vi "DAQ Mean Data UI.vi"() -> ()   [LabVIEW 2016]
uses:
  <vilib>/Utility/miscctls.llb/LVRowAndColumnTypeDef.ctl
  X-DAQ Viewer/Controls/ConfigFGVCtrl.ctl
  Ctrls/GlobeVaribles.vi
  Architecture/Queue Management/ARC_Queue Valid.vi
panel:
  out "Table":string[][](table)
  in  "Caller":string
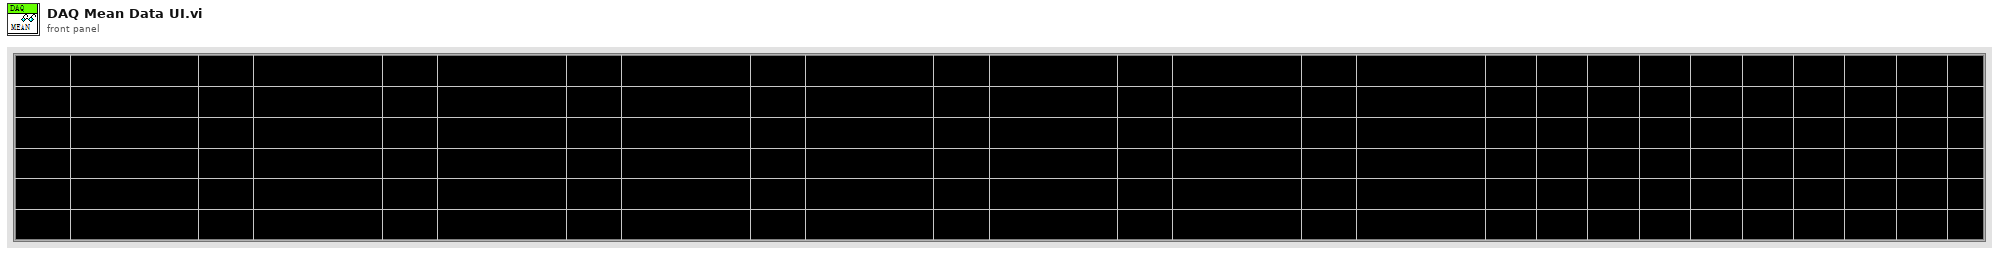
[diagram p1: front panel]
types:
  T1 = typedef "LVRowAndColumnTypeDef.ctl" = cluster{"Row":i32, "Column":i32}
  T2 = typedef "ConfigFGVCtrl.ctl" = enum16{"Initialize", "Get Value", "Set Value", "Search Info"}
  T3 = typedef "HardWare _ Channel Info.ctl" = cluster{"PhyCHtags[]":string[], "VCHTags":string[], "AllNames":string[], "AllAlias":string[], "AllUnits":string[], "AllName(Unit)":string[], "AllAlarmMax":dbl[], "AllAlarmMin":dbl[], "VCHFormula[]":string[], "VCHAlias[]":string[]}
  T4 = typedef "Continuous Operations.ctl" = enum16{"Writting", "Pause", "Stop"}
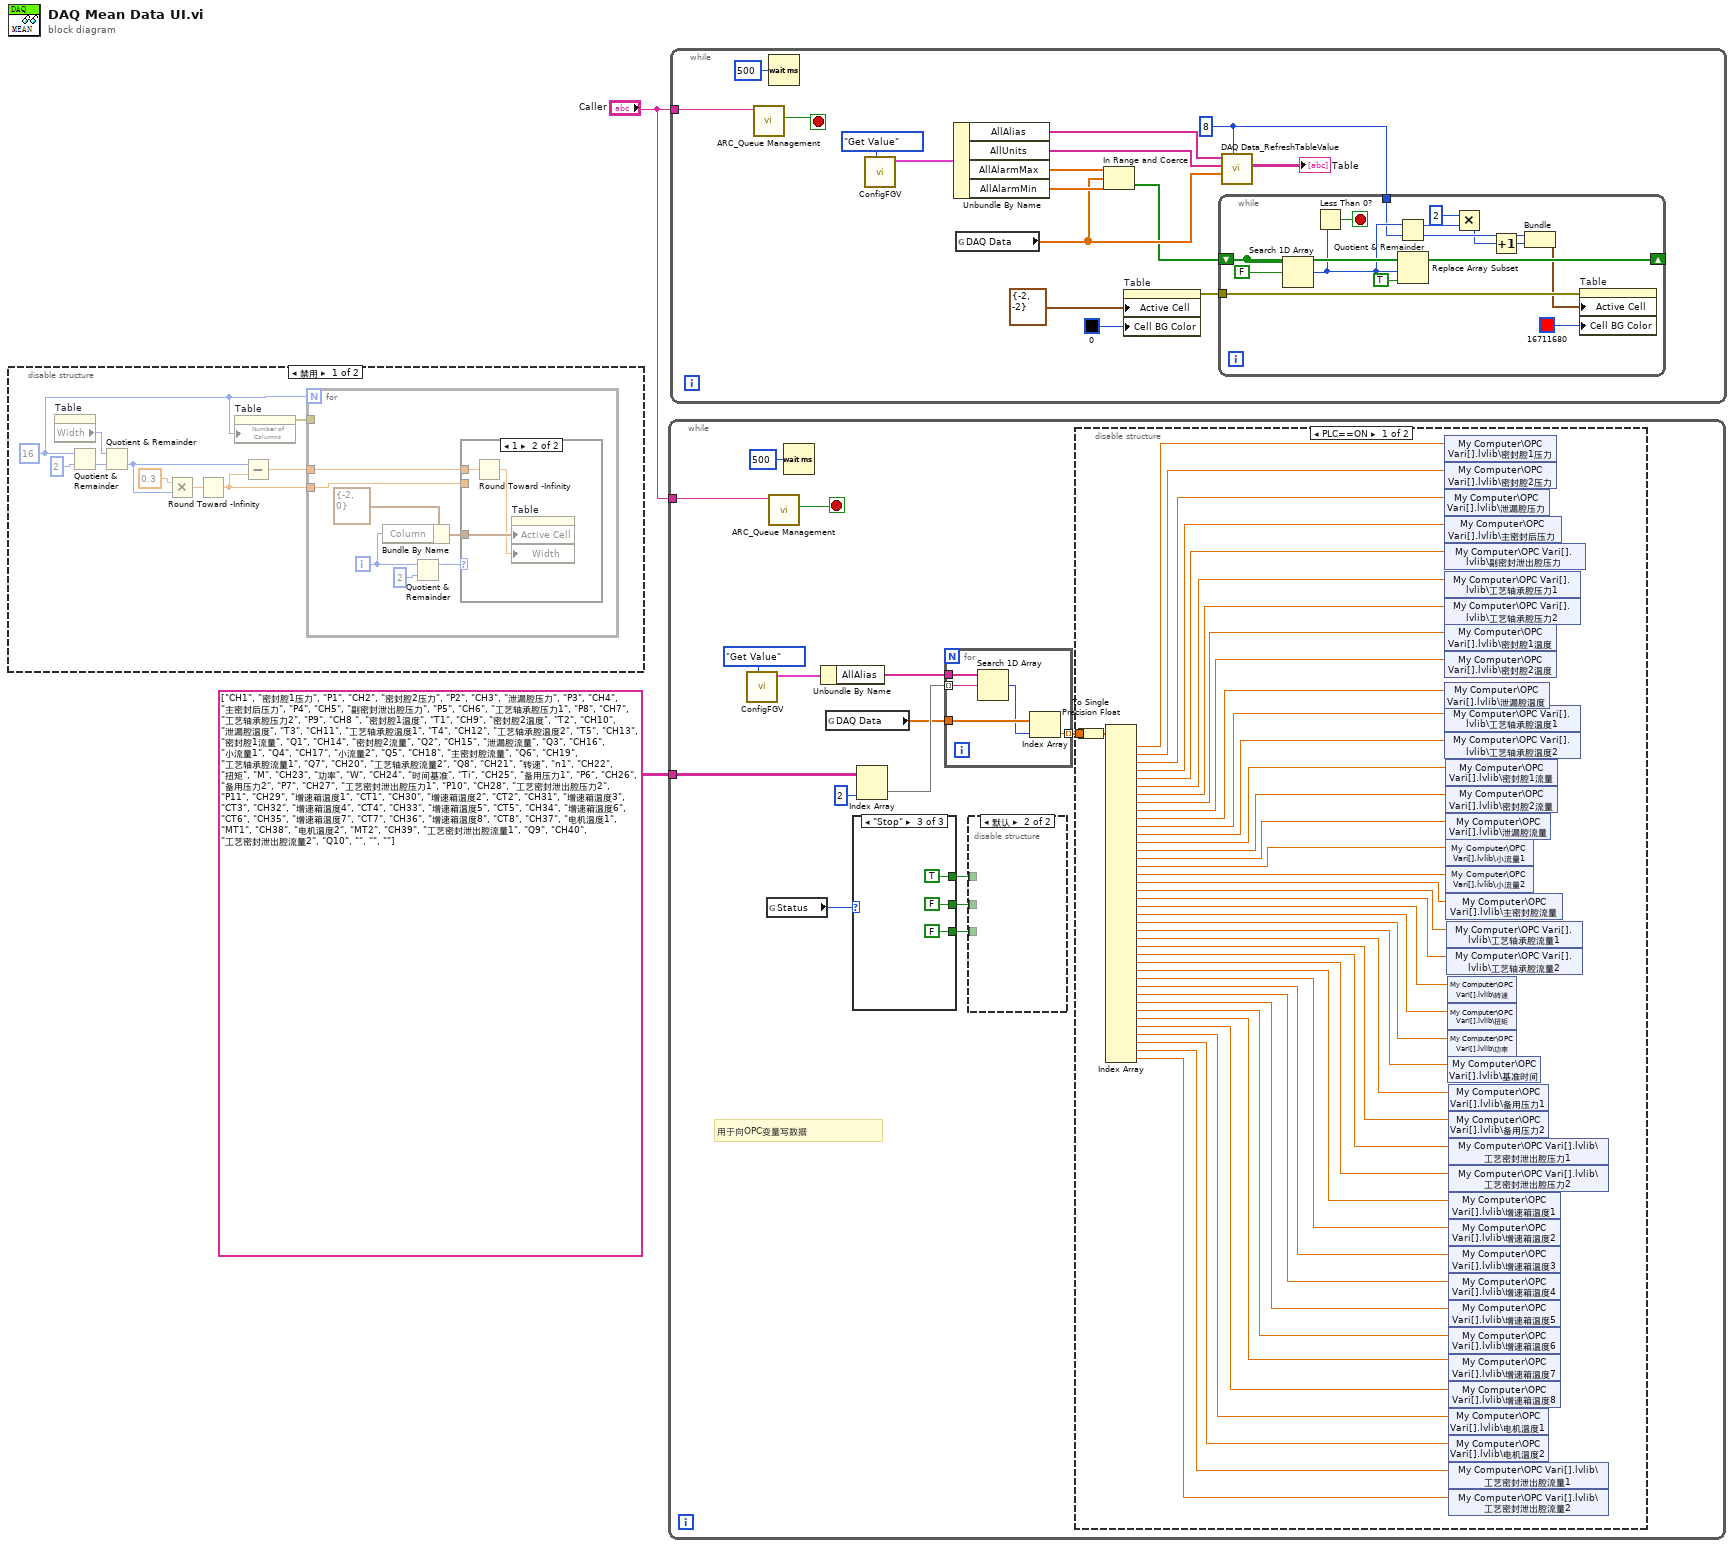
[diagram p0: block diagram]
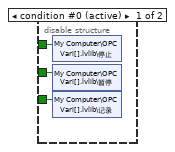
[diagram p2: hidden frame]
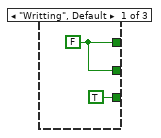
[diagram p4: hidden frame]
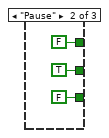
[diagram p5: hidden frame]
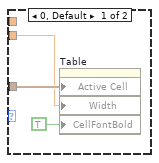
[diagram p6: hidden frame]
diagram:
  n1 = disable-structure shown="禁用" {
    frame Disabled {
      w4 = 16
      n2 = property on="Table" class="Tbl (strict)"() -> ("Width"=w9:u32)  [unwired: 2 in, 2 out]
      n3 = Quotient & Remainder(x=w4, y=2) -> (floor(x/y)=w11:i32)  [unwired: 1 out]
      n4 = Quotient & Remainder(x=w9, y=w11) -> (floor(x/y)=w6:u32)  [unwired: 1 out]
      n5 = Multiply(x=0.3, y=w6) -> (x*y=w8:dbl)
      n6 = Round Toward -Infinity(1:w8) -> (0:w5:dbl)
      n7 = property on="Table" class="Tbl (strict)"("Number of Columns"=w4) -> (error out=w3:errorcluster)  [unwired: 2 in, 1 out]
      n8 = Subtract(x=w6, y=w5) -> (x-y=w7:dbl)
      n9 = for {
        N: w4 -> [_]
        tunnel: w5 -> [w14]
        tunnel: w7 -> [w13]
        tunnel: w3 -> [_]
        i -> [w17]
        n10 = Bundle By Name(cluster=T1 {"Row"=-2, "Column"=0} ("活动单元格:活动单元格"), "Column"=w17) -> (w18:T1)
        n11 = Quotient & Remainder(x=w17, y=2) -> (x-y*floor(x/y)=w15:i32)  [unwired: 1 out]
        n12 = case shown="1" w15 {
          tunnel: w18 -> [w22 w25]
          tunnel: w14 -> [w20 _]
          tunnel: w13 -> [_ w24]
          frame 0, Default {
            n13 = property on="Table" class="Tbl (strict)"("Active Cell"=w22, "Width"=w20, "CellFontBold"=TRUE ("活动单元格:单元格字体:粗体")) -> ()  [unwired: 2 in, 2 out]
          }
          frame 1 {
            n14 = Round Toward -Infinity(1:w24) -> (0:w23:dbl)
            n15 = property on="Table" class="Tbl (strict)"("Active Cell"=w25, "Width"=w23) -> ()  [unwired: 2 in, 2 out]
          }
        }
      }
    }
    frame Enabled {
    }
  }
  n16 = while {
    tunnel: "Caller" -> [w39]
    tunnel: string[][] [["CH1", "密封腔1压力", "P1"], ["CH2", "密封腔2压力", "P2"], ["CH3", "泄漏腔压力", "P3"], ["CH4", "主密封后压力", "P4"], ["CH5", "副密封泄出腔压力", "P5"], ["CH6", "工艺轴承腔压力1", "P8"], ["CH7", "工艺轴承腔压力2", "P9"], ["CH8 ", "密封腔1温度", "T1"], ["CH9", "密封腔2温度", "T2"], ["CH10", "泄漏腔温度", "T3"], ["CH11", "工艺轴承腔温度1", "T4"], ["CH12", "工艺轴承腔温度2", "T5"], ["CH13", "密封腔1流量", "Q1"], ["CH14", "密封腔2流量", "Q2"], ["CH15", "泄漏腔流量", "Q3"], ["CH16", "小流量1", "Q4"], ["CH17", "小流量2", "Q5"], ["CH18", "主密封腔流量", "Q6"], ["CH19", "工艺轴承腔流量1", "Q7"], ["CH20", "工艺轴承腔流量2", "Q8"], ["CH21", "转速", "n1"], ["CH22", "扭矩", "M"], ["CH23", "功率", "W"], ["CH24", "时间基准", "Ti"], ["CH25", "备用压力1", "P6"], ["CH26", "备用压力2", "P7"], ["CH27", "工艺密封泄出腔压力1", "P10"], ["CH28", "工艺密封泄出腔压力2", "P11"], ["CH29", "增速箱温度1", "CT1"], ["CH30", "增速箱温度2", "CT2"], ["CH31", "增速箱温度3", "CT3"], ["CH32", "增速箱温度4", "CT4"], ["CH33", "增速箱温度5", "CT5"], ["CH34", "增速箱温度6", "CT6"], ["CH35", "增速箱温度7", "CT7"], ["CH36", "增速箱温度8", "CT8"], ["CH37", "电机温度1", "MT1"], ["CH38", "电机温度2", "MT2"], ["CH39", "工艺密封泄出腔流量1", "Q9"], ["CH40", "工艺密封泄出腔流量2", "Q10"], ["", "", ""]] ("数组") -> [w35]
    stop <- w38 stop-if-true
    # "用于向OPC变量写数据"
    n17 = call "ConfigFGV.vi"("Command"=ConfigFGVCtrl."Get Value") -> ("CHInfoOut"=w37:T3)  [unwired: 6 in, 4 out]
    n18 = global read "GlobeVaribles.vi" "Status"() -> (w29:T4)
    n19 = call-poly "ARC_Queue Management.vi"("Queue Name(unamed)"=w39) -> ("Not Exist?"=w38:bool)  [unwired: 8 in, 2 out]
    n20 = Wait (ms)(milliseconds to wait=u32 500 ("等待时间（毫秒）")) -> ()  [unwired: 1 out]
    n21 = Unbundle By Name(w37) -> ("AllAlias"=w33:string[])
    n22 = global read "GlobeVaribles.vi" "DAQ Data"() -> (w31:dbl[])
    n23 = case shown="\"Stop\"" w29 {
      tunnel: [w87 FALSE TRUE] -> w28
      tunnel: [w87 TRUE FALSE] -> w27
      tunnel: [TRUE FALSE FALSE] -> w26
      frame "Writting", Default {
        w87 = FALSE
      }
      frame "Pause" {
      }
      frame "Stop" {
      }
    }
    n24 = Index Array(array=w35, index (col)=2 ("禁用的索引 (列)")) -> (element=w32:string[])  [unwired: 1 in]
    n25 = for {
      tunnel: w33 -> [w98]
      tunnel: w32 -> [w97] mode=indexing
      tunnel: w31 -> [w96]
      tunnel: [w94] -> w30 mode=indexing
      n26 = Search 1D Array(1D array=w98, element=w97) -> (index of element=w95:i32)  [unwired: 1 in]
      n27 = Index Array(array=w96, index=w95) -> (element=w94:dbl)
    }
    n28 = disable-structure shown="默认" {
      disable-tunnel: w28 -> [w43 _]
      disable-tunnel: w27 -> [w42 _]
      disable-tunnel: w26 -> [w41 _]
      frame condition #0 (active) {
        n29 = shared-variable "My Computer\\OPC Vari[].lvlib\\停止"(w43) -> ()  [unwired: 1 in, 1 out]
        n30 = shared-variable "My Computer\\OPC Vari[].lvlib\\暂停"(w42) -> ()  [unwired: 1 in, 1 out]
        n31 = shared-variable "My Computer\\OPC Vari[].lvlib\\记录"(w41) -> ()  [unwired: 1 in, 1 out]
      }
      frame condition #1 {
      }
    }
    n32 = disable-structure shown="PLC==ON" {
      disable-tunnel: w30 -> [w85 _]
      frame condition #0 (active) {
        n33 = To Single Precision Float(number=w85) -> (single precision float=w79:sgl[])
        n34 = Index Array(array=w79) -> (element #1=w84:sgl, element #2=w83:sgl, element #3=w82:sgl, element #4=w81:sgl, element #5=w80:sgl, element #6=w78:sgl, element #7=w77:sgl, element #8=w76:sgl, element #9=w75:sgl, element #10=w74:sgl, element #11=w73:sgl, element #12=w72:sgl, element #13=w71:sgl, element #14=w70:sgl, element #15=w69:sgl, element #16=w68:sgl, element #17=w67:sgl, element #18=w66:sgl, element #19=w65:sgl, element #20=w64:sgl, element #21=w63:sgl, element #22=w62:sgl, element #23=w61:sgl, element #24=w44:sgl, element #25=w60:sgl, element #26=w59:sgl, element #27=w58:sgl, element #28=w57:sgl, element #29=w56:sgl, element #30=w55:sgl, element #31=w54:sgl, element #32=w53:sgl, element #33=w52:sgl, element #34=w51:sgl, element #35=w50:sgl, element #36=w49:sgl, element #37=w48:sgl, element #38=w47:sgl, element #39=w46:sgl, element #40=w45:sgl)  [unwired: 40 in]
        n35 = shared-variable "My Computer\\OPC Vari[].lvlib\\密封腔1压力"(w84) -> ()  [unwired: 1 in, 1 out]
        n36 = shared-variable "My Computer\\OPC Vari[].lvlib\\密封腔2压力"(w83) -> ()  [unwired: 1 in, 1 out]
        n37 = shared-variable "My Computer\\OPC Vari[].lvlib\\泄漏腔压力"(w82) -> ()  [unwired: 1 in, 1 out]
        n38 = shared-variable "My Computer\\OPC Vari[].lvlib\\主密封后压力"(w81) -> ()  [unwired: 1 in, 1 out]
        n39 = shared-variable "My Computer\\OPC Vari[].lvlib\\副密封泄出腔压力"(w80) -> ()  [unwired: 1 in, 1 out]
        n40 = shared-variable "My Computer\\OPC Vari[].lvlib\\工艺轴承腔压力1"(w78) -> ()  [unwired: 1 in, 1 out]
        n41 = shared-variable "My Computer\\OPC Vari[].lvlib\\工艺轴承腔压力2"(w77) -> ()  [unwired: 1 in, 1 out]
        n42 = shared-variable "My Computer\\OPC Vari[].lvlib\\密封腔1温度"(w76) -> ()  [unwired: 1 in, 1 out]
        n43 = shared-variable "My Computer\\OPC Vari[].lvlib\\密封腔2温度"(w75) -> ()  [unwired: 1 in, 1 out]
        n44 = shared-variable "My Computer\\OPC Vari[].lvlib\\泄漏腔温度"(w74) -> ()  [unwired: 1 in, 1 out]
        n45 = shared-variable "My Computer\\OPC Vari[].lvlib\\工艺轴承腔温度1"(w73) -> ()  [unwired: 1 in, 1 out]
        n46 = shared-variable "My Computer\\OPC Vari[].lvlib\\工艺轴承腔温度2"(w72) -> ()  [unwired: 1 in, 1 out]
        n47 = shared-variable "My Computer\\OPC Vari[].lvlib\\密封腔1流量"(w71) -> ()  [unwired: 1 in, 1 out]
        n48 = shared-variable "My Computer\\OPC Vari[].lvlib\\密封腔2流量"(w70) -> ()  [unwired: 1 in, 1 out]
        n49 = shared-variable "My Computer\\OPC Vari[].lvlib\\泄漏腔流量"(w69) -> ()  [unwired: 1 in, 1 out]
        n50 = shared-variable "My Computer\\OPC Vari[].lvlib\\小流量1"(w68) -> ()  [unwired: 1 in, 1 out]
        n51 = shared-variable "My Computer\\OPC Vari[].lvlib\\小流量2"(w67) -> ()  [unwired: 1 in, 1 out]
        n52 = shared-variable "My Computer\\OPC Vari[].lvlib\\主密封腔流量"(w66) -> ()  [unwired: 1 in, 1 out]
        n53 = shared-variable "My Computer\\OPC Vari[].lvlib\\工艺轴承腔流量1"(w65) -> ()  [unwired: 1 in, 1 out]
        n54 = shared-variable "My Computer\\OPC Vari[].lvlib\\工艺轴承腔流量2"(w64) -> ()  [unwired: 1 in, 1 out]
        n55 = shared-variable "My Computer\\OPC Vari[].lvlib\\转速"(w63) -> ()  [unwired: 1 in, 1 out]
        n56 = shared-variable "My Computer\\OPC Vari[].lvlib\\扭矩"(w62) -> ()  [unwired: 1 in, 1 out]
        n57 = shared-variable "My Computer\\OPC Vari[].lvlib\\功率"(w61) -> ()  [unwired: 1 in, 1 out]
        n58 = shared-variable "My Computer\\OPC Vari[].lvlib\\基准时间"(w44) -> ()  [unwired: 1 in, 1 out]
        n59 = shared-variable "My Computer\\OPC Vari[].lvlib\\备用压力1"(w60) -> ()  [unwired: 1 in, 1 out]
        n60 = shared-variable "My Computer\\OPC Vari[].lvlib\\备用压力2"(w59) -> ()  [unwired: 1 in, 1 out]
        n61 = shared-variable "My Computer\\OPC Vari[].lvlib\\工艺密封泄出腔压力1"(w58) -> ()  [unwired: 1 in, 1 out]
        n62 = shared-variable "My Computer\\OPC Vari[].lvlib\\工艺密封泄出腔压力2"(w57) -> ()  [unwired: 1 in, 1 out]
        n63 = shared-variable "My Computer\\OPC Vari[].lvlib\\增速箱温度1"(w56) -> ()  [unwired: 1 in, 1 out]
        n64 = shared-variable "My Computer\\OPC Vari[].lvlib\\增速箱温度2"(w55) -> ()  [unwired: 1 in, 1 out]
        n65 = shared-variable "My Computer\\OPC Vari[].lvlib\\增速箱温度3"(w54) -> ()  [unwired: 1 in, 1 out]
        n66 = shared-variable "My Computer\\OPC Vari[].lvlib\\增速箱温度4"(w53) -> ()  [unwired: 1 in, 1 out]
        n67 = shared-variable "My Computer\\OPC Vari[].lvlib\\增速箱温度5"(w52) -> ()  [unwired: 1 in, 1 out]
        n68 = shared-variable "My Computer\\OPC Vari[].lvlib\\增速箱温度6"(w51) -> ()  [unwired: 1 in, 1 out]
        n69 = shared-variable "My Computer\\OPC Vari[].lvlib\\增速箱温度7"(w50) -> ()  [unwired: 1 in, 1 out]
        n70 = shared-variable "My Computer\\OPC Vari[].lvlib\\增速箱温度8"(w49) -> ()  [unwired: 1 in, 1 out]
        n71 = shared-variable "My Computer\\OPC Vari[].lvlib\\电机温度1"(w48) -> ()  [unwired: 1 in, 1 out]
        n72 = shared-variable "My Computer\\OPC Vari[].lvlib\\电机温度2"(w47) -> ()  [unwired: 1 in, 1 out]
        n73 = shared-variable "My Computer\\OPC Vari[].lvlib\\工艺密封泄出腔流量1"(w46) -> ()  [unwired: 1 in, 1 out]
        n74 = shared-variable "My Computer\\OPC Vari[].lvlib\\工艺密封泄出腔流量2"(w45) -> ()  [unwired: 1 in, 1 out]
      }
      frame condition #1 {
      }
    }
  }
  n75 = while {
    tunnel: "Caller" -> [w113]
    stop <- w114 stop-if-true
    w99 = 8 ("前面板显示行数")
    n76 = call-poly "ARC_Queue Management.vi"("Queue Name(unamed)"=w113) -> ("Not Exist?"=w114:bool)  [unwired: 8 in, 2 out]
    n77 = Wait (ms)(milliseconds to wait=u32 500 ("等待时间（毫秒）")) -> ()  [unwired: 1 out]
    n78 = call "ConfigFGV.vi"("Command"=ConfigFGVCtrl."Get Value") -> ("CHInfoOut"=w110:T3)  [unwired: 6 in, 4 out]
    n79 = Unbundle By Name(w110) -> ("AllAlias"=w109:string[], "AllUnits"=w108:string[], "AllAlarmMax"=w106:dbl[], "AllAlarmMin"=w105:dbl[])
    n80 = global read "GlobeVaribles.vi" "DAQ Data"() -> (w104:dbl[])
    n81 = In Range and Coerce(upper limit=w106, x=w104, lower limit=w105) -> (In Range?=w103:bool[])  [unwired: 1 out]
    n82 = property on="Table" class="Tbl (strict)"("Active Cell"=T1 {"Row"=-2, "Column"=-2} ("活动单元格:活动单元格"), "Cell BG Color"=u32 0) -> (error out=w100:errorcluster)  [unwired: 2 in, 1 out]
    n83 = while {
      shift-right: [w126] -> _
      shift-left: w103 -> [w127]
      tunnel: w100 -> [w124]
      tunnel: w99 -> [w122]
      stop <- w128 stop-if-true
      n84 = Search 1D Array(1D array=w127, element=FALSE ("元素")) -> (index of element=w123:i32)  [unwired: 1 in]
      n85 = Less Than 0?(x=w123) -> (x < 0?=w128:bool)
      n86 = Quotient & Remainder(x=w123, y=w122) -> (x-y*floor(x/y)=w120:i32, floor(x/y)=w121:i32)
      n87 = Replace Array Subset(array=w127, new element=TRUE ("新元素/子数组"), index=w123) -> (w126:bool[])
      n88 = Multiply(x=2, y=w120) -> (x*y=w118:i32)
      n89 = Increment(x=w118) -> (x+1=w117:i32)
      n90 = Bundle(w121, w117) -> (w116:cluster{i32, i32})  [unwired: 1 in]
      n91 = property on="Table" class="Tbl (strict)"(error in=w124, "Active Cell"=w116, "Cell BG Color"=u32 16711680) -> ()  [unwired: 1 in, 2 out]
    }
    n92 = call "DAQ Data_RefreshTableValue.vi"("每行显示变量个数"=w99, "Data"=w104, "ChannelUnits"=w108, "ChannelNames"=w109) -> ("Table Data"=→"Table":string[][])  [unwired: 6 in, 1 out]
  }
